vi "NewLogReader.vi"() -> ()   [LabVIEW 2011]
doc: "Reads new (11-1-2012+) style logs and displays the data in a human-understandable format."
uses:
  0-OCU/0 Typedefs/Rudder Position.ctl
  2-Think/2 Typedefs/apparent wind direction.ctl
  2-Think/2 Typedefs/apparent wind speed.ctl
  2-Think/2 Typedefs/apparent wind.ctl
  2-Think/2 Typedefs/heading.ctl
  2-Think/2 Typedefs/UTM Location.ctl
  2-Think/2 Typedefs/robot velocity.ctl
  2-Think/2 Typedefs/pitch and roll.ctl
  0-OCU/0 Typedefs/Apparent Wind Point of Sail.ctl
  0-OCU/0 Typedefs/Maps.ctl
  0-OCU/0 Typedefs/Sail Position.ctl
  2-Think/2 Typedefs/UTM Circle.ctl
  <vilib>/vision/Image Controls.llb/IMAQ Image.ctl
  2-Think/2 Classes/Waypoint/Waypoint.lvclass
panel:
  in  "Choose graph to display":T1(tab)
  out "Rudder Manual?":bool
  out "Rudder Position":T2 scale=50.0..-50.0 scale format="%#_2f"
  out "Sail Manual?":bool
  in  "OCU":enum32{"Mission Map", "Detailed Telemetry"}(tab)
  out "Heading":T3 format="%05.1f"
  out "Goodness Functions Polar Plot":picture
  in  "Plot Colors":T4={"Target"=3381759, "No Sail"=16711680, "Change"=16756736, "Pure Waypt"=35080, "Pure Wind"=16860, "Combined"=16777228}
  out "Mission Map":T5(plugin-control)
  out "Apparent Wind Direction\nPoint of Sail":T6 scale=0.0..360.0 scale format="%4d"
  in  "Font Size":i16=40
  in  "Globals":enum32{"Where Am I", "What's Around Me"}(tab)
  out "Robot Heading":T3 format="%05.1f"
  out "Robot UTM Location":T7 {"North" format="%#_10f"; "East" format="%#_8f"}
  out "Robot Velocity":T8
  out "Robot Pitch/Roll":T9 {"Roll" format="%05.1f"; "Pitch" format="%05.1f"}
  out "Robot Speed (m/s)":dbl
  out "Apparent Wind Direction":T10
  out "Apparent Wind Speed":T11
  out "Apparent Wind":T12
  in  "Map Name":T13="LPB Pool"
  out "Sail Position":T14 scale=1.0..-1.0
  out "Location":cluster{dbl[], dbl[]}[](graph)
  out "Battery Voltage":cluster{i32[], dbl[]}(graph)
  out "Velocity":cluster{i32[], dbl[]}[](graph)
  out "Headings":cluster{i32[], dbl[]}[](graph)
  out "Rudder":cluster{i32[], dbl[]}(graph)
  out "Sail":cluster{i32[], dbl[]}(graph)
  in  "Time":i32(slide) max=625 scale=0.0..3415.0
  in  "stop":bool
  in  "Array":string[](array[string])=["RobotLocation", "RobotHeading", "RobotVelocity", "RobotPitch", "RobotRoll", "BatteryVoltage", "ApparentWindDirection", "ApparentWindSpeed", "Rudder", "Sail", "GoodnessFunctions", "NoSailZones", "Waypoint#", "WaypointTolerance", "WaypointCoordinates", "OverrideRudder", "OverrideSail"]
  out "Processing File....":path
  in  "Stop early":bool
  out "Percent Complete":u8(slide) scale=0.0..100.0
  # "As Measured"
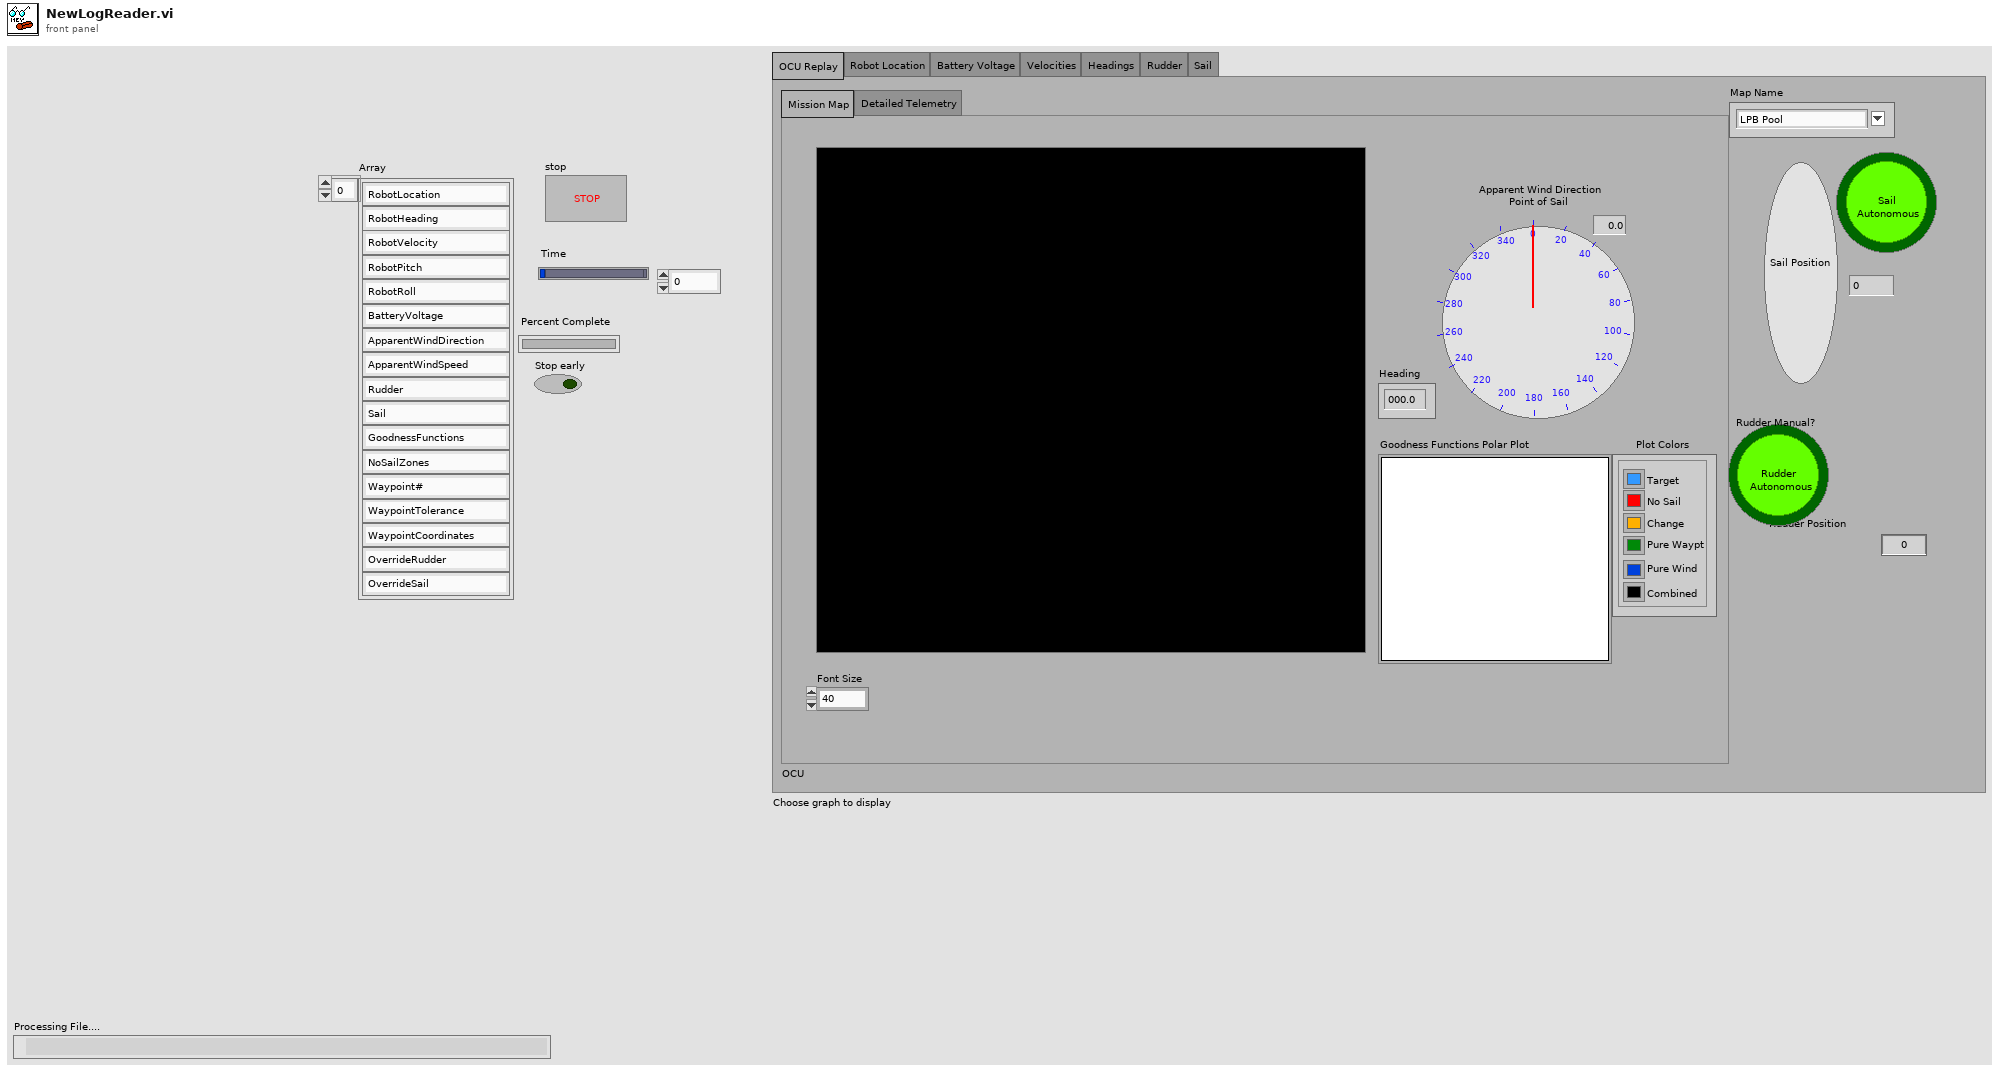
[diagram p1: front panel]
types:
  T1 = enum32{"OCU Replay", "Robot Location", "Battery Voltage", "Velocities", "Headings", "Rudder", "Sail"}
  T2 = typedef "Rudder Position.ctl" = dbl
  T3 = typedef "heading.ctl" = dbl
  T4 = cluster{"Target":u32, "No Sail":u32, "Change":u32, "Pure Waypt":u32, "Pure Wind":u32, "Combined":u32}
  T5 = typedef "IMAQ Image.ctl" = refnum<image>
  T6 = typedef "Apparent Wind Point of Sail.ctl" = dbl
  T7 = typedef "UTM Location.ctl" = cluster{"UTM Zone":dbl, "Hemisphere":enum16{"North", "South"}, "East":dbl, "North":dbl}
  T8 = typedef "robot velocity.ctl" = cluster{"East":dbl, "North":dbl}
  T9 = typedef "pitch and roll.ctl" = cluster{"Pitch":dbl, "Roll":dbl}
  T10 = typedef "apparent wind direction.ctl" = dbl
  T11 = typedef "apparent wind speed.ctl" = dbl
  T12 = typedef "apparent wind.ctl" = cluster{"Toward Fore":dbl, "Toward Starboard":dbl}
  T13 = typedef "Maps.ctl" = string
  T14 = typedef "Sail Position.ctl" = dbl
  T15 = typedef "UTM Circle.ctl" = cluster{"UTM Zone":dbl, "Hemisphere":enum16{"North", "South"}, "East":dbl, "North":dbl, "Radius":dbl}
  T16 = cluster{"RobotHeading":dbl, "RobotSpeed":dbl, "RobotPitch":dbl, "RobotRoll":dbl, "BatteryVoltage":dbl, "ApparentWindDirection":dbl, "ApparentWindSpeed":dbl, "Rudder":dbl, "Sail":dbl, "Waypoint#":dbl, "WaypointTolerance":dbl, "GoodnessFunctions":string, "OverrideRudder":bool, "OverrideSail":bool, "Global No Sail Circles":T15[], "Robot Location":T7, "WaypointCoordinates":T7}
  T17 = typedef "0-Image Descriptor.ctl" = cluster{"Upper-Left Corner Coordinates":T7, "Meters/Pixel":dbl}
  T18 = typedef "Velocity.ctl" = cluster{"East":dbl, "North":dbl}
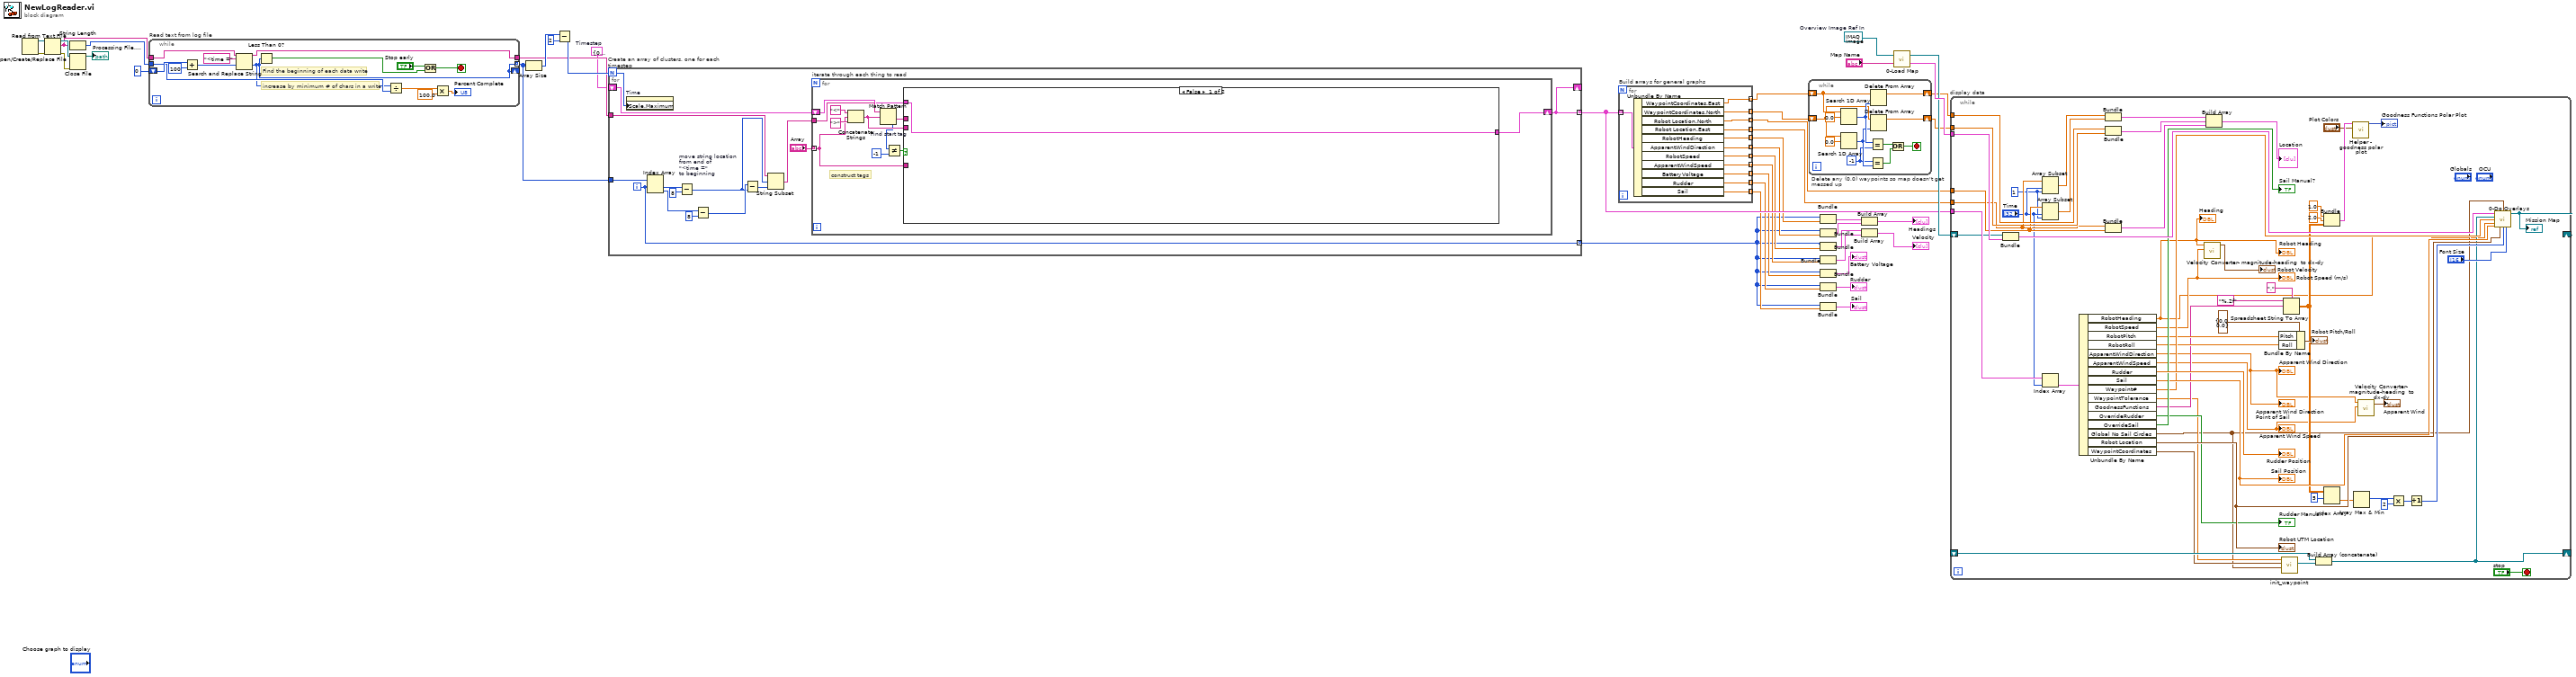
[diagram p0: block diagram]
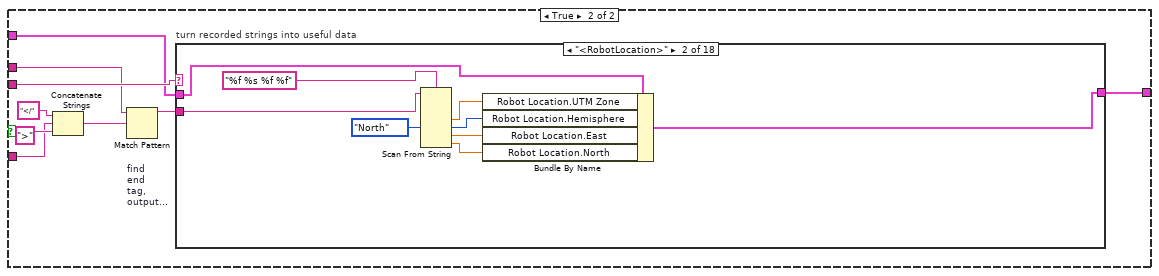
[diagram p2: hidden frame]
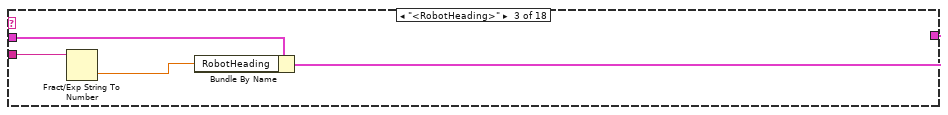
[diagram p4: hidden frame]
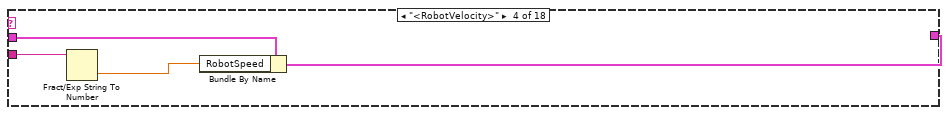
[diagram p5: hidden frame]
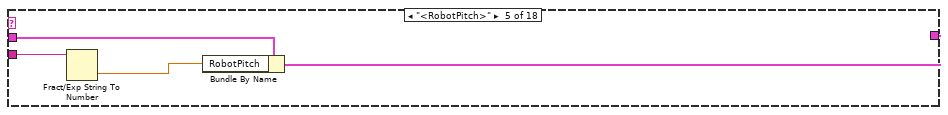
[diagram p6: hidden frame]
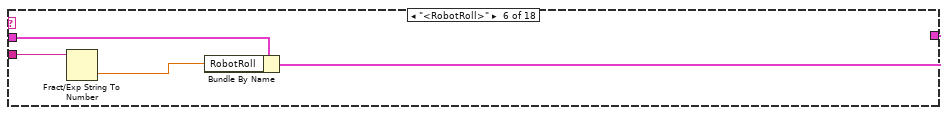
[diagram p7: hidden frame]
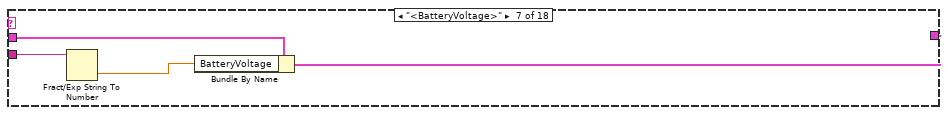
[diagram p8: hidden frame]
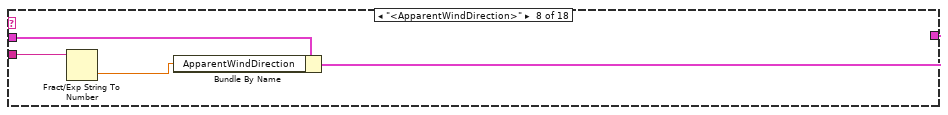
[diagram p9: hidden frame]
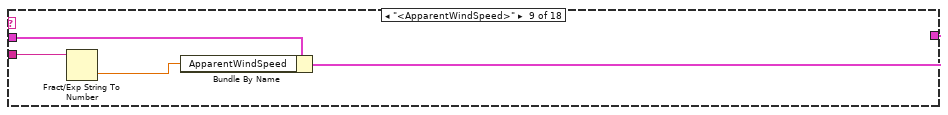
[diagram p10: hidden frame]
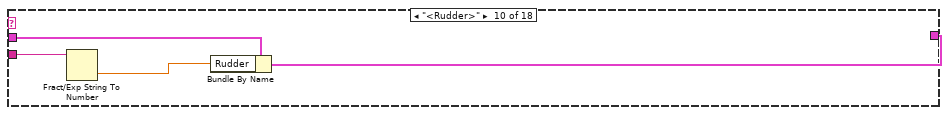
[diagram p11: hidden frame]
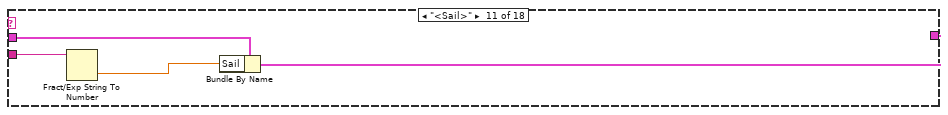
[diagram p12: hidden frame]
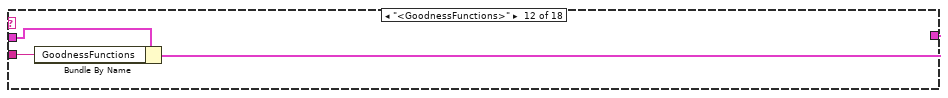
[diagram p13: hidden frame]
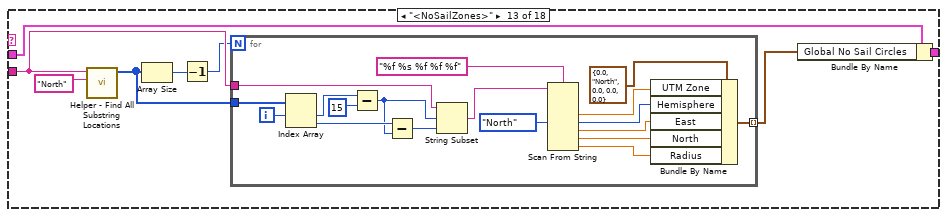
[diagram p14: hidden frame]
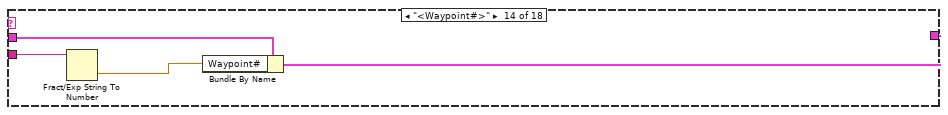
[diagram p15: hidden frame]
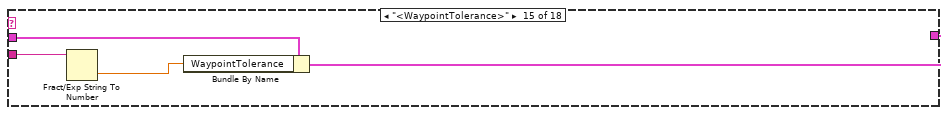
[diagram p16: hidden frame]
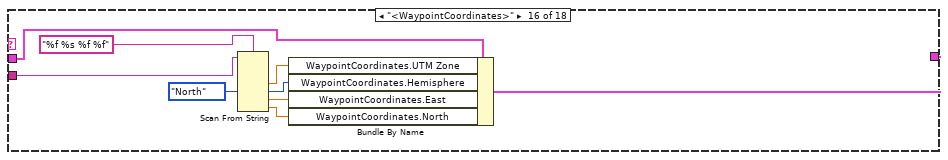
[diagram p17: hidden frame]
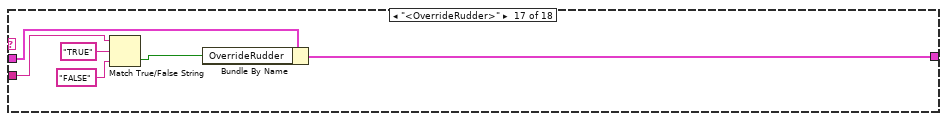
[diagram p18: hidden frame]
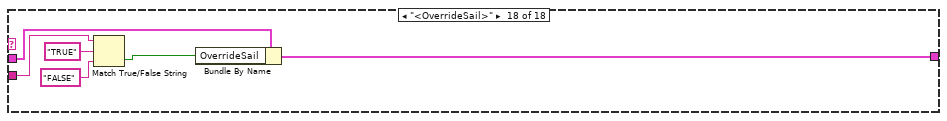
[diagram p19: hidden frame]
diagram:
  w28 = T5 refnum  # Overview Image Ref In
  w26 = T16 {"RobotHeading"=0.0, "RobotSpeed"=0.0, "RobotPitch"=0.0, "RobotRoll"=0.0, "BatteryVoltage"=0.0, "ApparentWindDirection"=0.0, "ApparentWindSpeed"=0.0, "Rudder"=0.0, "Sail"=0.0, "Waypoint#"=0.0, "WaypointTolerance"=0.0, "GoodnessFunctions"="", "OverrideRudder"=FALSE, "OverrideSail"=FALSE, "Global No Sail Circles"=[], "Robot Location"={"UTM Zone"=0.0, "Hemisphere"=enum."North", "East"=0.0, "North"=0.0}, "WaypointCoordinates"={"UTM Zone"=0.0, "Hemisphere"=enum."North", "East"=0.0, "North"=0.0}}  # Timestep
  n1 = Open/Create/Replace File() -> (refnum out=w42:refnum<file>, error out=w38:errorcluster)  [unwired: 6 in, 1 out]
  n2 = Read from Text File(file (use dialog)=w42, error in=w38) -> (refnum out=w39:refnum<file>, text=w36:string, error out=w40:errorcluster)  [unwired: 2 in, 1 out]
  n3 = String Length(string=w36) -> (length=w35:i32)
  n4 = Close File(refnum=w39, error in=w40) -> (path=→"Processing File....":path)  [unwired: 1 out]
  n5 = while "Read text from log file" {
    tunnel: w36 -> [w46]
    shift-right: [w44] -> _
    shift-left: 0 ("offset past replacement") -> [w56]
    tunnel: [w45] -> w30
    tunnel: [w44] -> w31 mode=indexing
    tunnel: w35 -> [w48]
    stop <- w54 stop-if-true
    # "increase by minimum # of chars in a write"
    # "Find the beginning of each data write"
    n6 = Add(x=w56, y=100) -> (x+y=w47:i32)
    n7 = Search and Replace String(input string=w46, search string="<time =", offset=w47) -> (result string=w45:string, offset past replacement=w44:i32)  [unwired: 5 in, 2 out]
    n8 = Less Than 0?(x=w44) -> (x < 0?=w52:bool)
    n9 = Divide(x=w44, y=w48) -> (x/y=w51:dbl)
    n10 = Or(x="Stop early", y=w52) -> (x .or. y?=w54:bool)
    n11 = Multiply(x=w51, y=100.0) -> (x*y=→"Percent Complete":dbl)
  }
  n12 = Array Size(array=w31) -> (size(s)=w34:i32)
  n13 = Subtract(x=w34, y=2) -> (x-y=w32:i32)
  n14 = for "Create an array of clusters, one for each timestep" {
    N: w32 -> [w62]
    tunnel: w31 -> [w71]
    tunnel: w30 -> [w66]
    tunnel: [w61] -> w24 mode=indexing
    shift-right: [w61] -> _
    shift-left: w26 -> [w60]
    tunnel: [w57] -> w5 mode=indexing
    i -> [w57]
    n15 = property on="Time" class="Slide (strict)"("Scale.Maximum"=w62) -> ()  [unwired: 2 in, 2 out]
    n16 = Index Array(array=w71, index #1=w57) -> (element #1=w70:i32, element #2=w67:i32)  [unwired: 1 in]
    n17 = Subtract "move string location\nfrom end of \n\"<time =\"\nto beginning"(x=w70, y=8) -> (x-y=w58:i32)
    n18 = Subtract(x=w67, y=8) -> (x-y=w59:i32)
    n19 = Subtract(x=w59, y=w58) -> (x-y=w65:i32)
    n20 = String Subset(string=w66, offset (0)=w58, length (rest)=w65) -> (substring=w64:string)
    n21 = for "iterate through each thing to read" {
      tunnel: w64 -> [w81]
      tunnel: "Array" -> [w79] mode=indexing
      shift-right: [w77] -> w61
      shift-left: w60 -> [w75]
      # "construct tags"
      n22 = Concatenate Strings("<" ("string"), w79, ">" ("string")) -> (w80:string)
      n23 = Match Pattern "Find start tag"(string=w81, regular expression=w80) -> (after substring=w76:string, offset past match=w73:i32)  [unwired: 1 in, 2 out]
      n24 = Not Equal?(x=w73, y=-1) -> (x != y?=w74:bool)
      n25 = case shown="False" w74 {
        tunnel: w80 -> [_ w89]
        tunnel: w79 -> [_ w88]
        tunnel: [w83 w87] -> w77
        tunnel: w76 -> [_ w85]
        tunnel: w75 -> [w83 w84]
        frame False {
        }
        frame True {
          n26 = Concatenate Strings("</" ("string"), w88, ">" ("string")) -> (w90:string)
          n27 = Match Pattern "find\nend\ntag,\noutput\nbetween\ntags"(string=w85, regular expression=w90) -> (before substring=w86:string)  [unwired: 1 in, 3 out]
          n28 = case "turn recorded strings into useful data" shown="\"<RobotLocation>\"" w89 {
            tunnel: w86 -> [_ w96 w106 w109 w112 w117 w119 w123 w127 w131 w135 w140 w147 w169 w172 w176 w185 w191]
            tunnel: w84 -> [w93 w98 w105 w110 w113 w116 w121 w125 w129 w133 w137 w141 w146 w170 w174 w183 w188 w193]
            tunnel: [w93 w97 w103 w107 w111 w115 w120 w124 w128 w132 w136 w139 w144 w168 w173 w179 w186 w192] -> w87
            frame Default {
              # "hopefully never needs to be used"
            }
            frame "<RobotLocation>" {
              n29 = Scan From String(format string="%f %s %f %f", input string=w96, default 2=enum16{"North", "South"}."North" ("Robot Location.Hemisphere")) -> (output 1=w101:dbl, output 2=w94:enum16{"North", "South"}, output 3=w100:dbl, output 4=w99:dbl)  [unwired: 5 in, 3 out]
              n30 = Bundle By Name(cluster=w98, "Robot Location.UTM Zone"=w101, "Robot Location.Hemisphere"=w94, "Robot Location.East"=w100, "Robot Location.North"=w99) -> (w97:T16)
            }
            frame "<RobotHeading>" {
              n31 = Fract/Exp String To Number(string=w106) -> (number=w104:dbl)  [unwired: 3 in, 1 out]
              n32 = Bundle By Name(cluster=w105, "RobotHeading"=w104) -> (w103:T16)
            }
            frame "<RobotVelocity>" {
              n33 = Fract/Exp String To Number(string=w109) -> (number=w108:dbl)  [unwired: 3 in, 1 out]
              n34 = Bundle By Name(cluster=w110, "RobotSpeed"=w108) -> (w107:T16)
            }
            frame "<RobotPitch>" {
              n35 = Fract/Exp String To Number(string=w112) -> (number=w114:dbl)  [unwired: 3 in, 1 out]
              n36 = Bundle By Name(cluster=w113, "RobotPitch"=w114) -> (w111:T16)
            }
            frame "<RobotRoll>" {
              n37 = Fract/Exp String To Number(string=w117) -> (number=w118:dbl)  [unwired: 3 in, 1 out]
              n38 = Bundle By Name(cluster=w116, "RobotRoll"=w118) -> (w115:T16)
            }
            frame "<BatteryVoltage>" {
              n39 = Fract/Exp String To Number(string=w119) -> (number=w122:dbl)  [unwired: 3 in, 1 out]
              n40 = Bundle By Name(cluster=w121, "BatteryVoltage"=w122) -> (w120:T16)
            }
            frame "<ApparentWindDirection>" {
              n41 = Fract/Exp String To Number(string=w123) -> (number=w126:dbl)  [unwired: 3 in, 1 out]
              n42 = Bundle By Name(cluster=w125, "ApparentWindDirection"=w126) -> (w124:T16)
            }
            frame "<ApparentWindSpeed>" {
              n43 = Fract/Exp String To Number(string=w127) -> (number=w130:dbl)  [unwired: 3 in, 1 out]
              n44 = Bundle By Name(cluster=w129, "ApparentWindSpeed"=w130) -> (w128:T16)
            }
            frame "<Rudder>" {
              n45 = Fract/Exp String To Number(string=w131) -> (number=w134:dbl)  [unwired: 3 in, 1 out]
              n46 = Bundle By Name(cluster=w133, "Rudder"=w134) -> (w132:T16)
            }
            frame "<Sail>" {
              n47 = Fract/Exp String To Number(string=w135) -> (number=w138:dbl)  [unwired: 3 in, 1 out]
              n48 = Bundle By Name(cluster=w137, "Sail"=w138) -> (w136:T16)
            }
            frame "<GoodnessFunctions>" {
              n49 = Bundle By Name(cluster=w141, "GoodnessFunctions"=w140) -> (w139:T16)
            }
            frame "<NoSailZones>" {
              n50 = call "Helper - Find All Substring Locations.vi"("search string"="North", "input string"=w147) -> ("Locations"=w148:i32[])  [unwired: 9 in]
              n51 = Array Size(array=w148) -> (size(s)=w142:i32)
              n52 = Decrement(x=w142) -> (x-1=w143:i32)
              n53 = for {
                N: w143 -> [_]
                tunnel: w148 -> [w167]
                tunnel: w147 -> [w164]
                tunnel: [w154] -> w145 mode=indexing
                i -> [w153]
                n54 = Index Array(array=w167, index #1=w153) -> (element #1=w152:i32, element #2=w151:i32)  [unwired: 1 in]
                n55 = Subtract(x=w152, y=15) -> (x-y=w150:i32)
                n56 = Subtract(x=w151, y=w150) -> (x-y=w165:i32)
                n57 = String Subset(string=w164, offset (0)=w150, length (rest)=w165) -> (substring=w163:string)
                n58 = Scan From String(format string="%f %s %f %f %f", input string=w163, default 2=enum16{"North", "South"}."North" ("Hemisphere")) -> (output 1=w160:dbl, output 2=w158:enum16{"North", "South"}, output 3=w157:dbl, output 4=w156:dbl, output 5=w155:dbl)  [unwired: 6 in, 3 out]
                n59 = Bundle By Name(cluster=T15 {"UTM Zone"=0.0, "Hemisphere"=enum."North", "East"=0.0, "North"=0.0, "Radius"=0.0} ("UTM Location"), "UTM Zone"=w160, "Hemisphere"=w158, "East"=w157, "North"=w156, "Radius"=w155) -> (w154:T15)
              }
              n60 = Bundle By Name(cluster=w146, "Global No Sail Circles"=w145) -> (w144:T16)
            }
            frame "<Waypoint#>" {
              n61 = Fract/Exp String To Number(string=w169) -> (number=w171:dbl)  [unwired: 3 in, 1 out]
              n62 = Bundle By Name(cluster=w170, "Waypoint#"=w171) -> (w168:T16)
            }
            frame "<WaypointTolerance>" {
              n63 = Fract/Exp String To Number(string=w172) -> (number=w175:dbl)  [unwired: 3 in, 1 out]
              n64 = Bundle By Name(cluster=w174, "WaypointTolerance"=w175) -> (w173:T16)
            }
            frame "<WaypointCoordinates>" {
              n65 = Scan From String(format string="%f %s %f %f", input string=w176, default 2=enum16{"North", "South"}."North" ("WaypointCoordinates.Hemisphere")) -> (output 1=w182:dbl, output 2=w177:enum16{"North", "South"}, output 3=w181:dbl, output 4=w180:dbl)  [unwired: 5 in, 3 out]
              n66 = Bundle By Name(cluster=w183, "WaypointCoordinates.UTM Zone"=w182, "WaypointCoordinates.Hemisphere"=w177, "WaypointCoordinates.East"=w181, "WaypointCoordinates.North"=w180) -> (w179:T16)
            }
            frame "<OverrideRudder>" {
              n67 = Match True/False String(2:"FALSE" ("false string"), 3:"TRUE" ("true string"), 4:w185) -> (0:w187:bool)  [unwired: 1 out]
              n68 = Bundle By Name(cluster=w188, "OverrideRudder"=w187) -> (w186:T16)
            }
            frame "<OverrideSail>" {
              n69 = Match True/False String(2:"FALSE" ("false string"), 3:"TRUE" ("true string"), 4:w191) -> (0:w194:bool)  [unwired: 1 out]
              n70 = Bundle By Name(cluster=w193, "OverrideSail"=w194) -> (w192:T16)
            }
          }
        }
      }
    }
  }
  n71 = for "Build arrays for general graphs" {
    tunnel: w24 -> [w208] mode=indexing
    tunnel: [w207] -> w20 mode=indexing
    tunnel: [w206] -> w19 mode=indexing
    tunnel: [w205] -> w10 mode=indexing
    tunnel: [w204] -> w9 mode=indexing
    tunnel: [w203] -> w7 mode=indexing
    tunnel: [w202] -> w6 mode=indexing
    tunnel: [w201] -> w2 mode=indexing
    tunnel: [w200] -> w1 mode=indexing
    tunnel: [w199] -> w3 mode=indexing
    tunnel: [w198] -> w4 mode=indexing
    tunnel: [w197] -> w8 mode=indexing
    n72 = Unbundle By Name(w208) -> ("WaypointCoordinates.East"=w201:dbl, "WaypointCoordinates.North"=w200:dbl, "Robot Location.North"=w199:dbl, "Robot Location.East"=w198:dbl, "RobotHeading"=w207:dbl, "ApparentWindDirection"=w206:dbl, "RobotSpeed"=w205:dbl, "ApparentWindSpeed"=w204:dbl, "BatteryVoltage"=w197:dbl, "Rudder"=w203:dbl, "Sail"=w202:dbl)
  }
  n73 = while "Delete any (0,0) waypoints so map doesn't get messed up" {
    shift-right: [w219] -> w12
    shift-left: w2 -> [w211]
    shift-right: [w209] -> w11
    shift-left: w1 -> [w210]
    stop <- w214 stop-if-true
    w215 = -1 ("y")
    n74 = Search 1D Array(1D array=w211, element=0.0) -> (index of element=w217:i32)  [unwired: 1 in]
    n75 = Search 1D Array(1D array=w210, element=0.0) -> (index of element=w216:i32)  [unwired: 1 in]
    n76 = Equal?(x=w217, y=w215) -> (x = y?=w213:bool)
    n77 = Equal?(x=w215, y=w216) -> (x = y?=w212:bool)
    n78 = Delete From Array(array=w211, index=w217) -> (array with subset deleted=w219:dbl[])  [unwired: 1 in, 1 out]
    n79 = Delete From Array(array=w210, index=w216) -> (array with subset deleted=w209:dbl[])  [unwired: 1 in, 1 out]
    n80 = Or(x=w213, y=w212) -> (x .or. y?=w214:bool)
  }
  n81 = Bundle(w5, w20) -> (w13:cluster{i32[], dbl[]})  [unwired: 1 in]
  n82 = Bundle(w5, w19) -> (w23:cluster{i32[], dbl[]})  [unwired: 1 in]
  n83 = Bundle(w5, w10) -> (w22:cluster{i32[], dbl[]})  [unwired: 1 in]
  n84 = Bundle(w5, w9) -> (w21:cluster{i32[], dbl[]})  [unwired: 1 in]
  n85 = Bundle(w5, w8) -> (→"Battery Voltage":cluster{i32[], dbl[]})  [unwired: 1 in]
  n86 = Bundle(w5, w7) -> (→"Rudder":cluster{i32[], dbl[]})  [unwired: 1 in]
  n87 = Bundle(w5, w6) -> (→"Sail":cluster{i32[], dbl[]})  [unwired: 1 in]
  n88 = Build Array(w13, w23) -> (→"Headings":cluster{i32[], dbl[]}[])
  n89 = Build Array(w22, w21) -> (→"Velocity":cluster{i32[], dbl[]}[])
  n90 = call "0-Load Map.vi"("Map Name"="Map Name", "Image Ref In"=w28) -> ("Image Descriptor"=w27:T17, "Image Ref Out"=w25:T5)
  n91 = while "display data" {
    tunnel: w24 -> [w276]
    tunnel: w27 -> [w273]
    shift-right: [w241] -> _
    shift-left: _ -> [w245]
    shift-right: [w240] -> _
    shift-left: w25 -> [w239]
    tunnel: w12 -> [w238]
    tunnel: w11 -> [w237]
    tunnel: w3 -> [w236]
    tunnel: w4 -> [w235]
    stop <- "stop" stop-if-true
    w233 = 1 ("length")
    n92 = Bundle("Image out"=w239, "Image Descriptor"=w273) -> (w272:cluster{"Image out":T5, "Image Descriptor":T17})  [unwired: 1 in]
    n93 = Array Subset(array=w235, index="Time", length=w233) -> (w232:dbl[])
    n94 = Array Subset(array=w236, index="Time", length=w233) -> (w231:dbl[])
    n95 = Index Array(array=w276, index="Time") -> (element=w275:T16)
    n96 = Unbundle By Name(w275) -> ("RobotHeading"=w225:dbl, "RobotSpeed"=w226:dbl, "RobotPitch"=w263:dbl, "RobotRoll"=w262:dbl, "ApparentWindDirection"=w222:dbl, "ApparentWindSpeed"=w221:dbl, "Rudder"=→"Rudder Position":dbl, "Sail"=w267:dbl, "Waypoint#"=w266:dbl, "WaypointTolerance"=w244:dbl, "GoodnessFunctions"=w260:string, "OverrideRudder"=→"Rudder Manual?":bool, "OverrideSail"=→"Sail Manual?":bool, "Global No Sail Circles"=w242:T15[], "Robot Location"=w270:T7, "WaypointCoordinates"=w243:T7)
    "Apparent Wind Direction\nPoint of Sail" <- w222
    "Heading" <- w225
    "Robot Speed (m/s)" <- w226
    "Robot Heading" <- w225
    "Sail Position" <- w267
    "Robot UTM Location" <- w270
    "Apparent Wind Direction" <- w222
    "Apparent Wind Speed" <- w221
    n97 = Bundle(w232, w231) -> (w230:cluster{dbl[], dbl[]})  [unwired: 1 in]
    n98 = Bundle(w238, w237) -> (w229:cluster{dbl[], dbl[]})  [unwired: 1 in]
    n99 = Bundle(w235, w236) -> (w228:cluster{dbl[], dbl[]})  [unwired: 1 in]
    n100 = call "Velocity Converter- magnitude-heading  to dx-dy.vi"("Magnitude"=w226, "Heading"=w225) -> ("Vector Out"=→"Robot Velocity":T18)  [unwired: 9 in]
    n101 = Build Array(w230, w229, w228) -> (→"Location":cluster{dbl[], dbl[]}[])
    n102 = Bundle By Name(cluster=T9 {"Pitch"=0.0, "Roll"=0.0} ("Robot Pitch/Roll"), "Pitch"=w263, "Roll"=w262) -> (→"Robot Pitch/Roll":T9)
    n103 = call "init_waypoint.vi"("No Sail Circles"=w242, "Coords"=w243, "Tolerance (m)"=w244) -> ("Waypoint Out"=w246:refnum<class "Waypoint.lvclass">)  [unwired: 8 in]
    n104 = Spreadsheet String To Array(delimiter (Tab)=",", format string="%.2f", spreadsheet string=w260) -> (array=w249:dbl[][])  [unwired: 1 in]
    n105 = Build Array (concatenate)(w245, w246) -> (w241:refnum<class "Waypoint.lvclass">[])
    n106 = Bundle(1.0, 2.0, w249) -> (w250:cluster{dbl, dbl, dbl[][]})  [unwired: 1 in]
    n107 = Index Array(array=w249, index (row)=5 ("disabled index (col)")) -> (element=w258:dbl[])  [unwired: 1 in]
    n108 = call "Helper - goodness polar plot.vi"("Plot Colors"="Plot Colors", "Goodness Fns In"=w250) -> ("Goodness Functions Polar Plot"=→"Goodness Functions Polar Plot":picture)  [unwired: 9 in]
    n109 = Array Max & Min(array=w258) -> (max index (indices)=w257:i32)  [unwired: 3 out]
    n110 = call "Velocity Converter- magnitude-heading  to dx-dy.vi"("Magnitude"=w221, "Heading"=w222) -> ("Vector Out"=→"Apparent Wind":T18)  [unwired: 9 in]
    n111 = Multiply(x=w257, y=2) -> (x*y=w255:i32)
    n112 = Increment(x=w255) -> (x+1=w253:i32)
    n113 = call "0-Do Overlays.vi"("Image Reference\nand Descriptor"=w272, "No Sail Circles"=w242, "Waypoints"=w241, "Current Waypoint #"=w266, "Heading"=w225, "Sail Position"=w267, "Robot UTM Location"=w270, "Optimal Heading"=w253, "Font Size"="Font Size") -> ("Image out"=w240:T5)  [unwired: 6 in]
    "Mission Map" <- w240
  }
